vi "PH_Cont-601k_PSU.PC Remote Controlled.vi"(0 "i ref in":refnum<vi>, 5 "error in (no error)":errorcluster) -> (14 "i ref out":refnum<vi>, 19 "error out":errorcluster)   [LabVIEW 2014, in "PH_Cont-601k_PSU.lvlib"]
doc: "This is the Proc Case \"Remote Control\"."
uses:
  PH_Cont-601k_PSU.lvlib
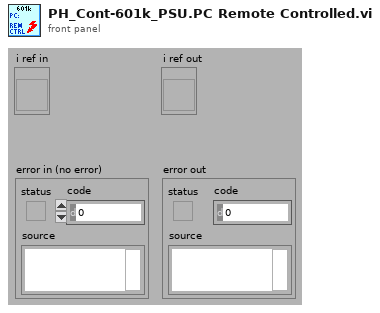
[diagram p1: front panel]
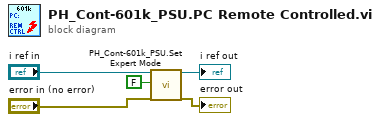
[diagram p0: block diagram]
diagram:
  n1 = call "PH_Cont-601k_PSU.Set Expert Mode.vi"("VI in"="i ref in", "Expert working"=FALSE, "error in (no error)"="error in (no error)") -> ("VI out"=→"i ref out":refnum<vi>, "error out"=→"error out":errorcluster)  [unwired: 15 in]
